vi "Service Mode Test Select.vi"(0 "GEA2 Reference In":refnum<k24>, 5 "High\\Low End":enum16{"HE", "LE"}(ring), 7 "Test Number In":T1=enum."Test 1 - Fault Codes", 11 "Error In":errorcluster) -> (4 "GEA2 Reference Out":refnum<k24>, 15 "Error Out":errorcluster)   [LabVIEW 2016, in "Centauro.lvlib"]
uses:
  Projects/Centauro.lvlib
  Q:/Common/DLLs/GEA3/GeaCommunication.dll
  Common/DLLs/GEA3/GeaCommunication.dll
  type defs/Service mode Tests.ctl
  Common/LabVIEW GEA2 Toolkit/LabVIEW_GEA2_Toolkit.lvlibp/type defs/Source_Destination.ctl
  type defs/Service Mode Pointer.ctl
  Common/LabVIEW GEA2 Toolkit/LabVIEW_GEA2_Toolkit.lvlibp
panel:
  in  "Standalone?":bool
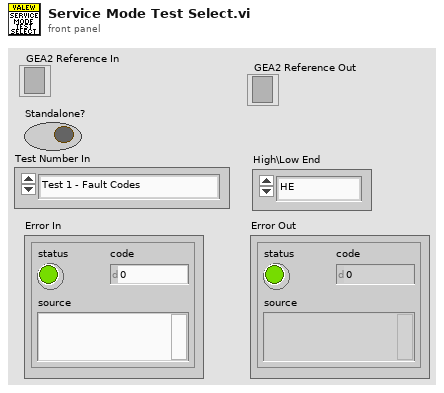
[diagram p1: front panel]
types:
  T1 = typedef "Centauro.lvlib/Service mode Tests.ctl" = enum16{"Test 0 - All LEDs on", "Test 1 - Fault Codes", "Test 2 - Personality ID", "Test 3 - MC Software Ver(Crit)", "Test 4 -MC Software Ver(Non-crit)", "Test 5 - XML Ver (Non-Crit) ", "Test 6 - UI Software Ver(Crit)", "Test 7 - UI Software Ver (Non-Crit)", "Test 8 - Hot Water Valve", "Test 9 - Cold Water Valve", "Test 10 - Pressure Sensor", "Test 11 - Drain Pump", "Test 12 - Lid Switch", "Test 13 -Spin", "Test 14 - Agitate", "Test 15 - Clear all Fcodes", "Test 16 - Analog Knob"}
  T2 = typedef "LabVIEW_GEA2_Toolkit.lvlibp/Source_Destination.ctl" = cluster{"Source":u8, "Destination":u8}
  T3 = typedef "Service Mode Pointer.ctl" = enum16{"Set ", "Get"}
  T4 = enum16{"CycleKnobPosition0", "CycleKnobPosition1", "CycleKnobPosition2", "CycleKnobPosition3", "CycleKnobPosition4", "CycleKnobPosition5", "CycleKnobPosition6", "CycleKnobPosition7", "CycleKnobPosition8", "CycleKnobPosition9", "CycleKnobPosition10", "CycleKnobPosition11"}
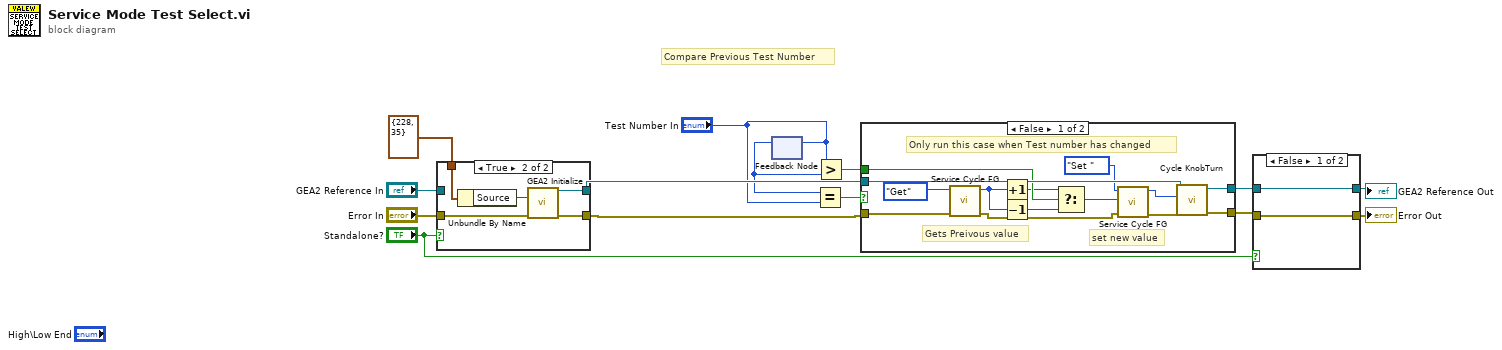
[diagram p0: block diagram]
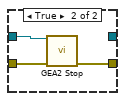
[diagram p3: hidden frame]
diagram:
  # "Compare Previous Test Number"
  n1 = case shown="True" "Standalone?" {
    tunnel: "Error In" -> [w15 w21]
    tunnel: [w15 w20] -> w5
    tunnel: "GEA2 Reference In" -> [w16 _]
    tunnel: [w16 w19] -> w8
    tunnel: T2 {"Source"=228, "Destination"=35} ("GEA Inputs") -> [_ w17]
    frame False {
    }
    frame True {
      n2 = Unbundle By Name(w17) -> ("Source"=w18:u8)
      n3 = call "GEA2 Initialize.vi"("Source Address"=w18, "error in"=w21) -> ("GEA2 Reference Out"=w19:refnum<k24>, "error out"=w20:errorcluster)  [unwired: 11 in, 1 out]
    }
  }
  n4 = feedback-in #1("Test Number In") -> ()
  n5 = feedback #1() -> (w3:T1)  [unwired: 1 in]
  n6 = Equal?(x=w3, y="Test Number In") -> (x = y?=w1:bool)
  n7 = Greater?(x="Test Number In", y=w3) -> (0:w4:bool)
  n8 = case shown="False" w1 {
    tunnel: w8 -> [w35 w37]
    tunnel: [w34 w37] -> w7
    tunnel: [w33 w36] -> w6
    tunnel: w5 -> [w31 w36]
    tunnel: w4 -> [w30 _]
    frame False {
      # "Only run this case when Test number has changed"
      # "Gets Preivous value"
      # "set new value"
      n9 = call "Service Cycle FG.vi"("Error In"=w31, "Action"=Service_Mode_Pointer."Get") -> ("Error Out"=w25:errorcluster, "Cycle Knob Out"=w28:T4)  [unwired: 8 in]
      n10 = Increment(x=w28) -> (x+1=w29:T4)
      n11 = Decrement(x=w28) -> (x-1=w27:T4)
      n12 = Select(t=w29, s=w30, f=w27) -> (s? t:f=w22:T4)
      n13 = call "Service Cycle FG.vi"("Error In"=w25, "Cycle Knob"=w22, "Action"=Service_Mode_Pointer."Set ") -> ("Error Out"=w26:errorcluster, "Cycle Knob Out"=w24:T4)  [unwired: 7 in]
      n14 = call "Cycle KnobTurn.vi"("Error In"=w26, "Cycle Knob"=w24, "GEA2 Reference In"=w35) -> ("Error Out"=w33:errorcluster, "GEA2 Reference Out"=w34:refnum<k24>)  [unwired: 7 in]
    }
    frame True {
      # "If previous test number is equal do nothing"
    }
  }
  n15 = case shown="False" "Standalone?" {
    tunnel: [w38 w42] -> w12
    tunnel: w7 -> [w39 w41]
    tunnel: [w39 _] -> w9
    tunnel: w6 -> [w38 w40]
    frame False {
    }
    frame True {
      n16 = call "GEA2 Stop.vi"("GEA2 Reference In"=w41, "Error In"=w40) -> ("Error Out"=w42:errorcluster)  [unwired: 13 in]
    }
  }
  "Error Out" <- w12
  "GEA2 Reference Out" <- w9
